vi "Destroy User Event - Stop.vi"(8 "entrée d'erreur (pas d'erreur)":errorcluster, 11 "Événement utilisateur - Arrêt":refnum<user-event>) -> (0 "sortie d'erreur":errorcluster)   [LabVIEW 2016, in "User Event - Stop.lvlib"]
doc: "Supprimer l'événement utilisateur, même s'il y a une erreur en entrée."
uses:
  User Event - Stop.lvlib
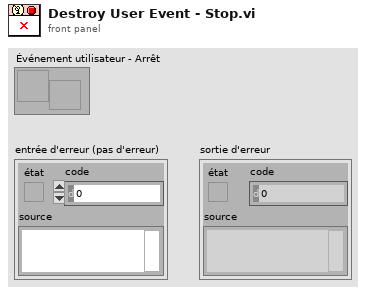
[diagram p1: front panel]
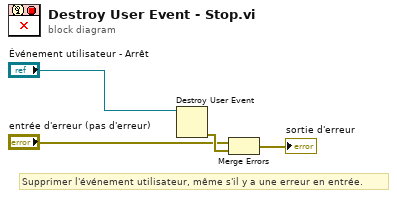
[diagram p0: block diagram]
diagram:
  # "Supprimer l'événement utilisateur, même s'il y a une erreur en entrée."
  n1 = Destroy User Event(user event="Événement utilisateur - Arrêt") -> (error out=w3:errorcluster)  [unwired: 1 in]
  n2 = Merge Errors("entrée d'erreur (pas d'erreur)", w3) -> (→"sortie d'erreur":errorcluster)
